vi "Profiled_PID_DriveFwdBck_Example.vi"() -> ()   [LabVIEW 2019]
uses:
  <vilib>/Rock Robotics/WPI/ThirdParty/JAS_Junk/TrajLib/ProfiledPIDController_SetPID.vi
  <vilib>/Rock Robotics/WPI/ThirdParty/JAS_Junk/TrajLib/ProfiledPIDController_SetIntegratorRange.vi
  <vilib>/Rock Robotics/WPI/ThirdParty/JAS_Junk/TrajLib/ProfiledPIDController_SetTolerance_PosVel.vi
  <vilib>/Rock Robotics/WPI/ThirdParty/JAS_Junk/TrajLib/ProfiledPIDController_DisableContInput.vi
  <vilib>/Rock Robotics/WPI/ThirdParty/JAS_Junk/TrajLib/ProfiledPIDController_EnableContInput.vi
  <vilib>/Rock Robotics/WPI/ThirdParty/JAS_Junk/TrajLib/ProfiledPIDController_Reset_PosOnly.vi
  <vilib>/Rock Robotics/WPI/ThirdParty/JAS_Junk/TrajLib/ProfiledPIDController_NewPeriod.vi
  <vilib>/Rock Robotics/WPI/ThirdParty/JAS_Junk/TrajLib/ProfiledPIDController_Calculate_Meas_Goal.vi
  <vilib>/Rock Robotics/WPI/ThirdParty/JAS_Junk/TrajLib/ProfiledPIDController_AtGoal.vi
  <vilib>/Rock Robotics/WPI/ThirdParty/JAS_Junk/TrajLib/ProfiledPIDController_AtSetpoint.vi
  <vilib>/Rock Robotics/WPI/ThirdParty/JAS_Junk/TrajLib/ProfiledPIDController_SetConstraints.vi
  <vilib>/Rock Robotics/WPI/ThirdParty/JAS_Junk/TrajLib/PIDController_GetVelocityError.vi
  <vilib>/Rock Robotics/WPI/ThirdParty/JAS_Junk/TrajLib/PIDController_GetPositionError.vi
  <vilib>/Rock Robotics/WPI/ThirdParty/JAS_Junk/TrajLib/PIDController_SetPID.vi
  <vilib>/Rock Robotics/WPI/ThirdParty/JAS_Junk/TrajLib/PIDController_SetIntegratorRange.vi
  <vilib>/Rock Robotics/WPI/ThirdParty/JAS_Junk/TrajLib/PIDController_SetTolerancePandV.vi
  <vilib>/Rock Robotics/WPI/ThirdParty/JAS_Junk/TrajLib/PIDController_DisableContinousInput.vi
  <vilib>/Rock Robotics/WPI/ThirdParty/JAS_Junk/TrajLib/PIDController_EnableContinousInput.vi
  <vilib>/Rock Robotics/WPI/ThirdParty/JAS_Junk/TrajLib/TrapProfState_New.vi
  <vilib>/Rock Robotics/WPI/ThirdParty/JAS_Junk/TrajLib/ProfiledPIDController_Reset.vi
  <vilib>/Rock Robotics/WPI/ThirdParty/JAS_Junk/TrajLib/PIDController_NewPeriod.vi
  <vilib>/Rock Robotics/SystemInterfaces/NetworkCommunication/NetComm_UsageReport_report.vi
  <vilib>/Rock Robotics/WPI/ThirdParty/JAS_Junk/TrajLib/ProfiledPIDController_SetGoal_PosOnly.vi
  <vilib>/Rock Robotics/WPI/ThirdParty/JAS_Junk/TrajLib/ProfiledPIDController_Calculate_Meas.vi
  <vilib>/Rock Robotics/WPI/ThirdParty/JAS_Junk/TrajLib/TrapProfState_Equals.vi
  <vilib>/Rock Robotics/WPI/ThirdParty/JAS_Junk/TrajLib/PIDController_AtSetpoint.vi
  <vilib>/Rock Robotics/WPI/ThirdParty/JAS_Junk/TrajLib/PIDController_Reset.vi
  <vilib>/Rock Robotics/WPI/ThirdParty/JAS_Junk/TrajLib/ProfiledPIDController_SetGoal.vi
  <vilib>/Rock Robotics/WPI/ThirdParty/JAS_Junk/TrajLib/PIDController_Calculate_SP_PV.vi
  <vilib>/Rock Robotics/WPI/ThirdParty/JAS_Junk/TrajLib/TrapProfile_New.vi
  <vilib>/Rock Robotics/WPI/ThirdParty/JAS_Junk/TrajLib/ProfiledPIDController_GetPeriod.vi
  <vilib>/Rock Robotics/WPI/ThirdParty/JAS_Junk/TrajLib/TrapProfile_Calculate.vi
  <vilib>/Rock Robotics/WPI/ThirdParty/JAS_Junk/TrajLib/ControllerUtil_GetModulusError.vi
  <vilib>/Rock Robotics/WPI/ThirdParty/JAS_Junk/TrajLib/PIDController_SetSetpoint.vi
  <vilib>/Rock Robotics/WPI/ThirdParty/JAS_Junk/TrajLib/PIDController_Calculate_PV.vi
  <vilib>/Rock Robotics/WPI/ThirdParty/JAS_Junk/TrajLib/TrapProfile_ShouldFlipAcceleration.vi
  <vilib>/Rock Robotics/WPI/ThirdParty/JAS_Junk/TrajLib/TrapProfile_Direct.vi
  <vilib>/Rock Robotics/WPI/ThirdParty/JAS_Junk/TrajLib/PIDController_GetPeriod.vi
  <vilib>/Rock Robotics/WPI/ThirdParty/JAS_Junk/TrajLib/Util_LibraryGlobals.vi
  <vilib>/Rock Robotics/WPI/ThirdParty/JAS_Junk/TrajLib/Trajectory_Library.lvlib
panel:
  in  "Tab Control":enum32{"Operation", "Tuning"}(tab)
  out "Targets along the way":T1(graph)
  in  "SP - Desired Position\n (Inch)":dbl(slide) scale=-10.0..350.0
  out "PV - Current Position\n (Inch)":dbl(slide) scale=-10.0..350.0
  out "Goal":T2(graph)
  out "Motor Output":dbl format="%13.3f"
  out "AtSetpoint":bool
  out "AtGoal":bool
  out "PositionError  \n(Inch)":dbl format="%13.2f"
  out "VelocityError  \n(Inch/Sec)":dbl format="%13.2f"
  out "Velocity  (Inch/Sec)":dbl format="%13.2f"
  out "Velocity  \n(Inch/Sec) 2":dbl format="%13.2f"
  in  "Kp":dbl=0.08 format="%#_13g"
  in  "Ki":dbl=0.15 format="%#_13g"
  in  "Kd":dbl format="%#_13g"
  in  "Minimum Integral":dbl=-0.3 format="%#_13g"
  in  "Maximum Integral":dbl=0.3 format="%#_13g"
  in  "Max Speed   (Inch/Sec)":dbl=84.0 format="%#_13g"
  in  "Max Accel  (Inch/Sec^2)":dbl=60.0 format="%#_13g"
  in  "PositionTolerance\n(Inch)":dbl=0.08 format="%#_13g"
  in  "VelocityTolerance\n(Inch/Sec)":dbl=0.01 format="%#_13g"
  # "Position has hard limit\n at -5 and 300 inches"
  # "SET THESE BEFORE EXECUTING THIS PROGRAM."
  # "PID Tuning Parameters"
  # "Desired Profile Performance"
  # "Desired On Target Tolerance"
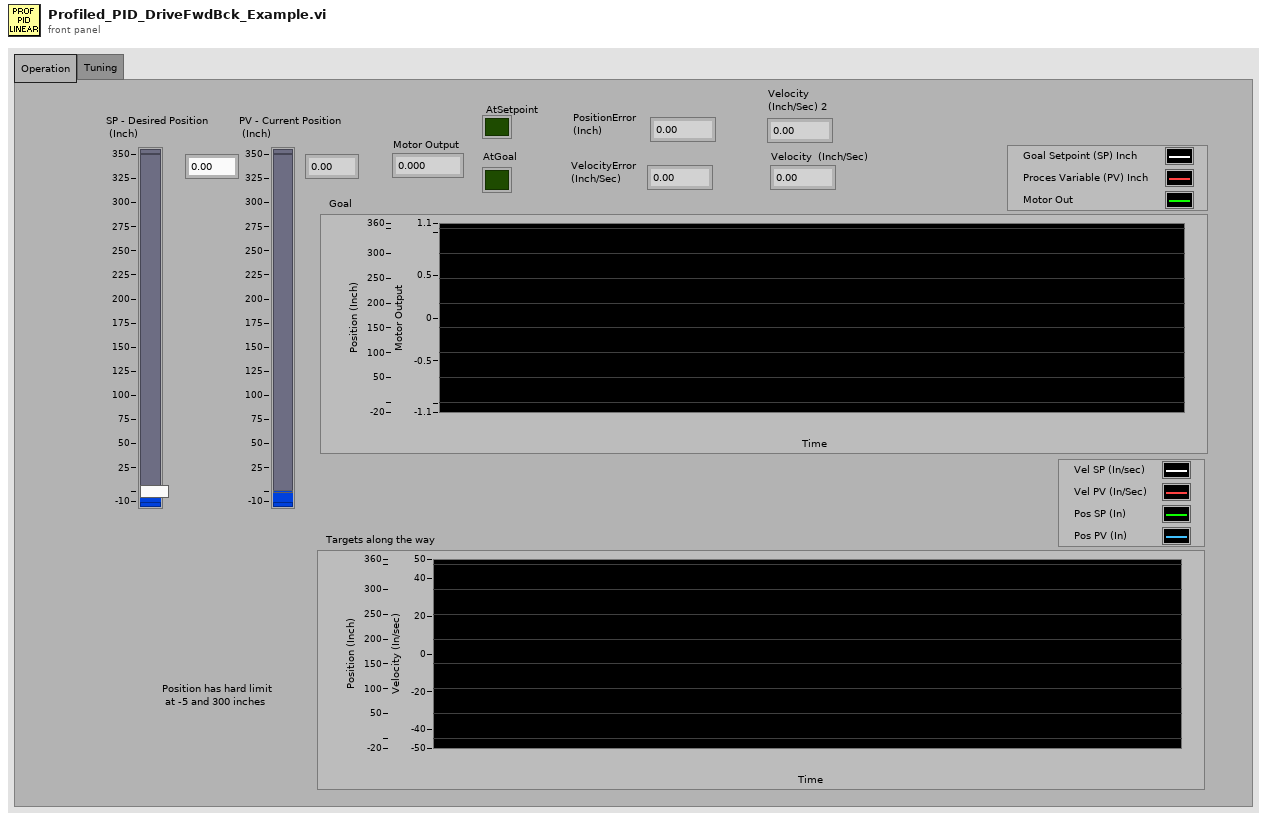
[diagram p1: front panel]
types:
  T1 = cluster{"SP - Desired Heading\n (Deg)":dbl, "PV - Current Heading\n (Deg)":dbl, "upper limit":dbl, dbl}
  T2 = cluster{"SP - Desired Position\n (Inch)":dbl, "upper limit":dbl, "upper limit":dbl}
  T3 = typedef "Trajectory_Library.lvlib/PID_TUNING.ctl" = cluster{"Kp":dbl, "Ki":dbl, "Kd":dbl, "MaximumIntegral":dbl, "MinimumIntegral":dbl}
  T4 = typedef "Trajectory_Library.lvlib/PID_ERROR_TOLERANCE.ctl" = cluster{"PositionTolerance":dbl, "VelocityTolerance":dbl}
  T5 = typedef "Trajectory_Library.lvlib/PID_INPUT_LIMITS.ctl" = cluster{"MaxInput":dbl, "MinInput":dbl, "Continuous":bool}
  T6 = typedef "Trajectory_Library.lvlib/TRAPEZOID_PROFILE_CONSTRAINT.ctl" = cluster{"MaxVelocity":dbl, "MaxAcceleration":dbl}
  T7 = typedef "Trajectory_Library.lvlib/PROFILED_PID_CONTROLLER.ctl" = cluster{"Controller":T8, "Goal":T9, "Setpoint":T9, "Constraint":T6}
  T8 = typedef "Trajectory_Library.lvlib/PID_CONTROLLER.ctl" = cluster{"Kp":dbl, "Ki":dbl, "Kd":dbl, "Period":dbl, "Max_Integral":dbl, "Min_Integral":dbl, "Max_Input":dbl, "Min_Input":dbl, "Continuous":bool, "PositionError":dbl, "VelocityError":dbl, "PrevError":dbl, "TotalError":dbl, "PositionTolerance":dbl, "VelocityTolerance":dbl, "SetPoint":dbl, "Kf":dbl, "Prev_Deriv":dbl, "Prev_Deriv 2":dbl, "DerivativeFilter":bool, "Min_Output":dbl, "Max_Output":dbl, "Prev_F_P":dbl, "Prev_F_P_2":dbl, "AntiWindupActive":bool, "Measurement":dbl}
  T9 = typedef "Trajectory_Library.lvlib/TRAPEZOID_PROFILE_STATE.ctl" = cluster{"Position":dbl, "Velocity":dbl}
  T10 = cluster{"Velocity":dbl, dbl, "Position":dbl, dbl}
  T11 = cluster{"SP - Desired Position\n (Inch)":dbl, dbl, "Result":dbl}
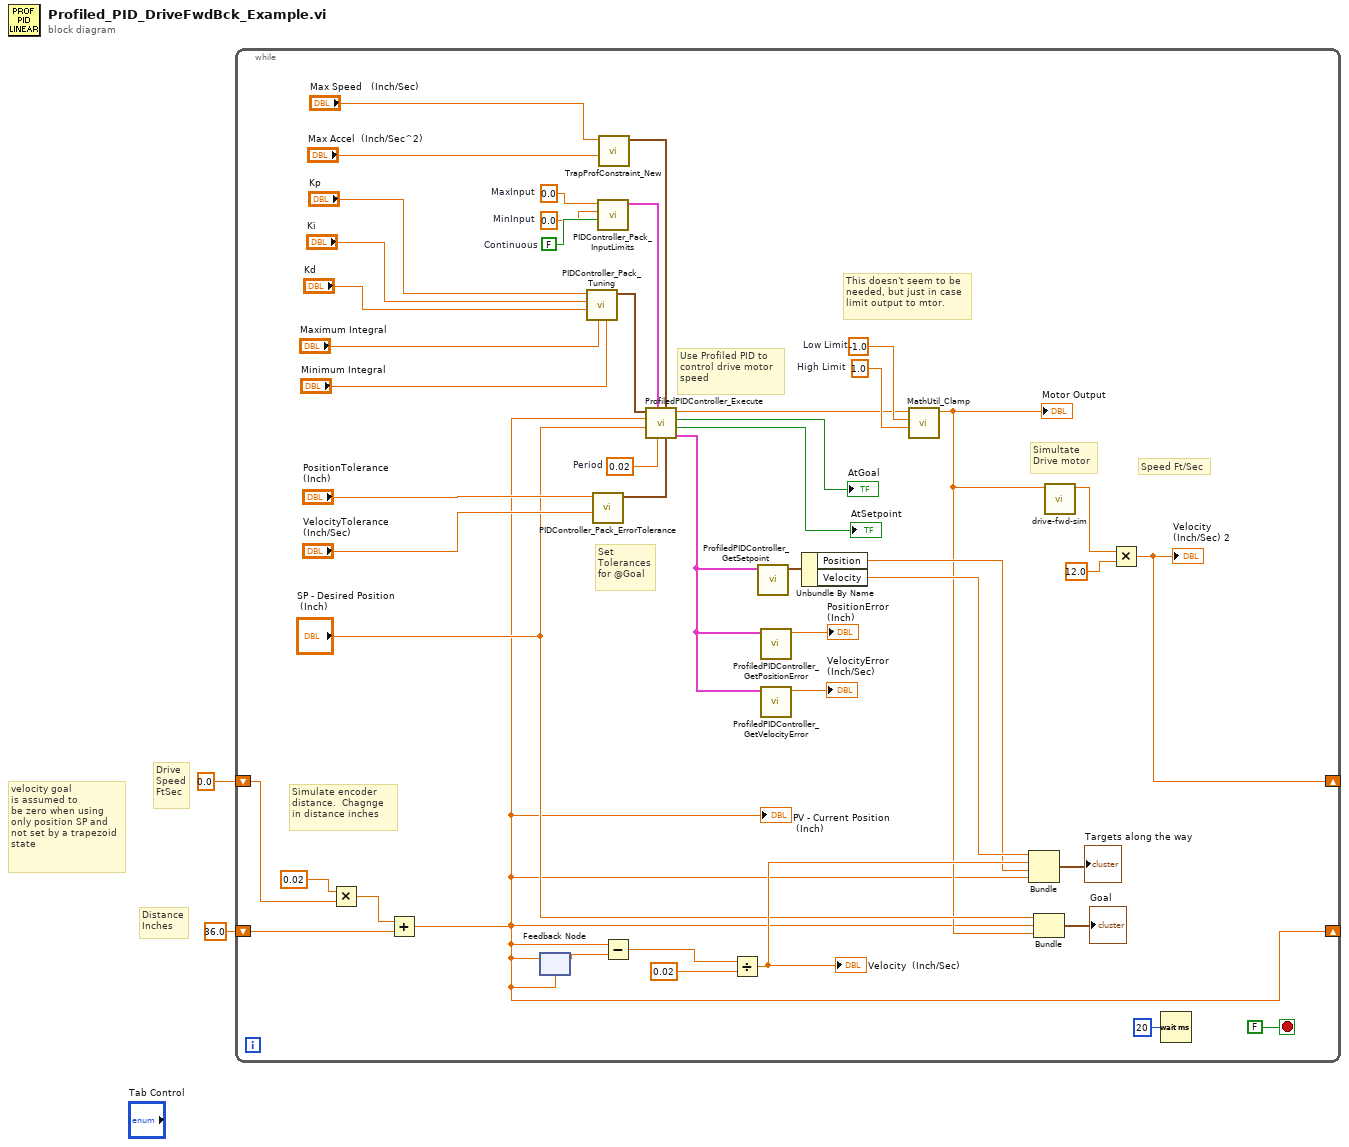
[diagram p0: block diagram]
diagram:
  # "velocity goal\nis assumed to \nbe zero when using\nonly position SP and\nnot set by a trapezoid\nstate"
  # "Distance\nInches"
  # "Drive\nSpeed\nFtSec"
  n1 = while {
    shift-right: [w4] -> _
    shift-left: 36.0 ("upper limit") -> [w38]
    shift-right: [w5] -> _
    shift-left: 0.0 ("upper limit") -> [w12]
    stop <- FALSE stop-if-true
    w11 = 1.0  # High Limit
    w10 = -1.0  # Low Limit
    w16 = 0.0  # MaxInput
    w17 = 0.0  # MinInput
    w18 = FALSE  # Continuous
    w19 = 0.02  # Period
    # "This doesn't seem to be\nneeded, but just in case\nlimit output to mtor."
    # "Use Profiled PID to\ncontrol drive motor\nspeed"
    # "Speed Ft/Sec"
    # "Simultate \nDrive motor"
    # "Simulate encoder \ndistance.  Chagnge \nin distance inches"
    # "Set\nTolerances\nfor @Goal"
    n2 = Multiply(x=0.02 ("value"), y=w12) -> (x*y=w40:dbl)
    n3 = Add(x=w40, y=w38) -> (x+y=w4:dbl)
    "PV - Current Position\n (Inch)" <- w4
    n4 = feedback-in #1(w4) -> ()
    n5 = feedback #1(w4) -> (w46:dbl)
    n6 = call <vilib>:"PIDController_Pack_Tuning.vi"("MinimumIntegral"="Minimum Integral", "MaximumIntegral"="Maximum Integral", "Kd"="Kd", "Ki"="Ki", "Kp"="Kp") -> ("PID Tuning"=w21:T3)  [unwired: 6 in]
    n7 = call <vilib>:"PIDController_Pack_ErrorTolerance.vi"("VelocityTolerance"="VelocityTolerance\n(Inch/Sec)", "PositionTolerance"="PositionTolerance\n(Inch)") -> ("PID Error Tolerance"=w30:T4)  [unwired: 9 in]
    n8 = call <vilib>:"PIDController_Pack_InputLimits.vi"("Continuous"=w18, "MinInput"=w17, "MaxInput"=w16) -> ("PID Input Limits"=w22:T5)  [unwired: 8 in]
    n9 = call <vilib>:"TrapProfConstraint_New.vi"("Max Accel"="Max Accel  (Inch/Sec^2)", "Max Speed (M/S)"="Max Speed   (Inch/Sec)") -> ("TRAPEZOID_PROFILE_CONSTRAINT"=w20:T6)  [unwired: 9 in]
    n10 = Subtract(x=w4, y=w46) -> (x-y=w45:dbl)
    n11 = call <vilib>:"ProfiledPIDController_Execute.vi"("PID Error Tolerance"=w30, "Constraints"=w20, "Period"=w19, "PID Input Limits"=w22, "SP-SetPoint Goal"="SP - Desired Position\n (Inch)", "PV-Measurement"=w4, "PID Tuning"=w21) -> ("out PID_CONTROLLER"=w3:T7, "AtSetpoint"=→"AtSetpoint":bool, "AtGoal"=→"AtGoal":bool, "CO-ControlOutput"=w9:dbl)  [unwired: 1 in]
    n12 = Divide(x=w45, y=0.02) -> (x/y=w34:dbl)
    "Velocity  (Inch/Sec)" <- w34
    n13 = call <vilib>:"ProfiledPIDController_GetSetpoint.vi"("in PROFILED_PID_CONTROLLER"=w3) -> ("Setpoint"=w36:T9)  [unwired: 10 in]
    n14 = call <vilib>:"ProfiledPIDController_GetPositionError.vi"("in PROFILED_PID_CONTROLLER"=w3) -> ("PositionError"=→"PositionError  \n(Inch)":dbl)  [unwired: 10 in]
    n15 = call <vilib>:"ProfiledPIDController_GetVelocityError.vi"("in PROFILED_PID_CONTROLLER"=w3) -> ("VelocityError"=→"VelocityError  \n(Inch/Sec)":dbl)  [unwired: 10 in]
    n16 = Unbundle By Name(w36) -> ("Position"=w33:dbl, "Velocity"=w35:dbl)
    n17 = call <vilib>:"MathUtil_Clamp.vi"("High Limit"=w11, "Low Limit"=w10, "Value"=w9) -> ("Result"=w8:dbl)  [unwired: 8 in]
    "Motor Output" <- w8
    n18 = Bundle("Velocity"=w35, w34, "Position"=w33, w4) -> (→"Targets along the way":T10)  [unwired: 1 in]
    n19 = Bundle("SP - Desired Position\n (Inch)"="SP - Desired Position\n (Inch)", w4, "Result"=w8) -> (→"Goal":T11)  [unwired: 1 in]
    n20 = call "drive-fwd-sim.vi"("Motor Demand"=w8) -> ("Drive Speed Ft/Sec"=w7:dbl)  [unwired: 10 in]
    n21 = Multiply(x=w7, y=12.0) -> (x*y=w5:dbl)
    "Velocity  \n(Inch/Sec) 2" <- w5
    n22 = Wait (ms)(milliseconds to wait=u32 20) -> ()  [unwired: 1 out]
  }
